vi "tabbed result string.vi"() -> (1 "read success":bool, 2 "tabbed string":string)   [LabVIEW 2010]
uses:
  serial commands.ctl
panel:
  out "Read line":string
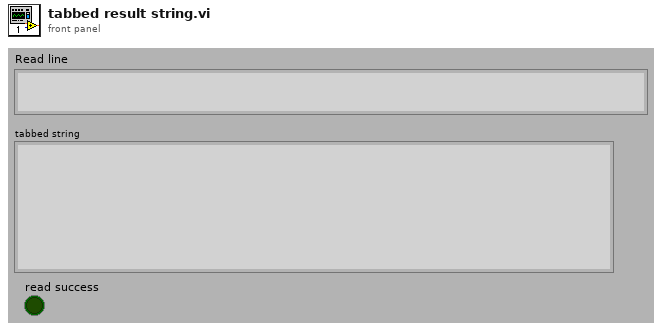
[diagram p1: front panel]
types:
  T1 = typedef "serial commands.ctl" = enum16{"configure", "VISA resource", "write line", "read line", "Clear buffer", "close"}
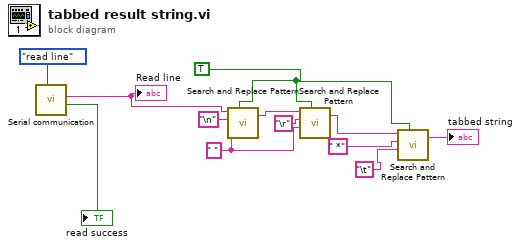
[diagram p0: block diagram]
diagram:
  w4 = " " ("replace string (\"\")")
  w6 = TRUE ("replace all? (F)")
  n1 = call <userlib>:"Serial communication.vi"("serial commands"=serial_commands."read line") -> ("read success"=→"read success":bool, "Read line"=w2:string)  [unwired: 4 in, 2 out]
  "Read line" <- w2
  n2 = call <vilib>:"Search and Replace Pattern.vi"("string"=w2, "regular expression (\"\")"="\n" ("regular expression (\"\")"), "replace string (\"\")"=w4, "replace all? (F)"=w6) -> ("result string"=w7:string)  [unwired: 1 in, 1 out]
  n3 = call <vilib>:"Search and Replace Pattern.vi"("string"=w7, "regular expression (\"\")"="\r" ("regular expression (\"\")"), "replace string (\"\")"=w4, "replace all? (F)"=w6) -> ("result string"=w3:string)  [unwired: 1 in, 1 out]
  n4 = call <vilib>:"Search and Replace Pattern.vi"("string"=w3, "regular expression (\"\")"=" *" ("search string"), "replace string (\"\")"="\t" ("replace string (\"\")"), "replace all? (F)"=w6) -> ("result string"=→"tabbed string":string)  [unwired: 1 in, 1 out]
